vi "Add Percent Codes.vi"(11 "String":string) -> (3 "String 2":string)   [LabVIEW 2020]
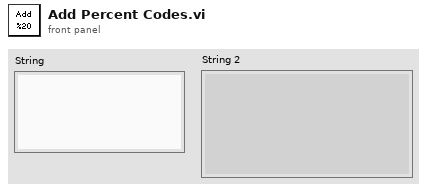
[diagram p1: front panel]
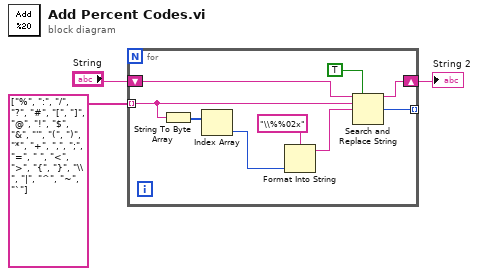
[diagram p0: block diagram]
diagram:
  n1 = for {
    tunnel: string[] ["%", ":", "/", "?", "#", "[", "]", "@", "!", "$", "&", "'", "(", ")", "*", "+", ",", ";", "=", " ", "<", ">", "{", "}", "\\", "|", "^", "~", "`"] -> [w12] mode=indexing
    shift-right: [w6] -> w1
    shift-left: "String" -> [w7]
    tunnel: [w4] -> _ mode=indexing
    n2 = String To Byte Array(string=w12) -> (unsigned byte array=w11:u8[])
    n3 = Index Array(array=w11) -> (element=w10:u8)  [unwired: 1 in]
    n4 = Format Into String(format string="\\%%02x", w10) -> (resulting string=w8:string)  [unwired: 2 in, 1 out]
    n5 = Search and Replace String(replace all?=TRUE ("replace all? (F)"), input string=w7, search string=w12, replace string=w8) -> (result string=w6:string, number of replacements=w4:i32)  [unwired: 4 in, 2 out]
  }
  "String 2" <- w1
